vi "crc16-ccitt (xFFFF).vi"(8 "error in (no error)":errorcluster, 10 "Message":string) -> (0 "error out (dup)":errorcluster, 2 "CRC":u16 format="%.0x")   [LabVIEW 2017]
doc: "This VI takes in a string variable and calculates the 16-bit CRC value based on the CRC16-CCITT standard (polynomial 0x1021) with seed value of 0xFFFF ONLY!!!\n\nThis VI code is based on an extremely efficient implementation originally intended for microcontrollers and is adapted for LabVIEW. All thanks go to:\nOriginal Code: Ashley Roll\nOptimisations: Scott Dattalo"
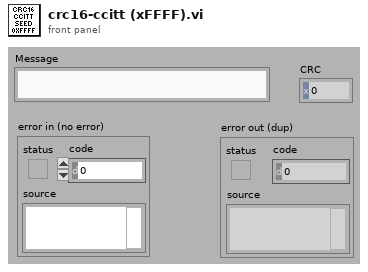
[diagram p1: front panel]
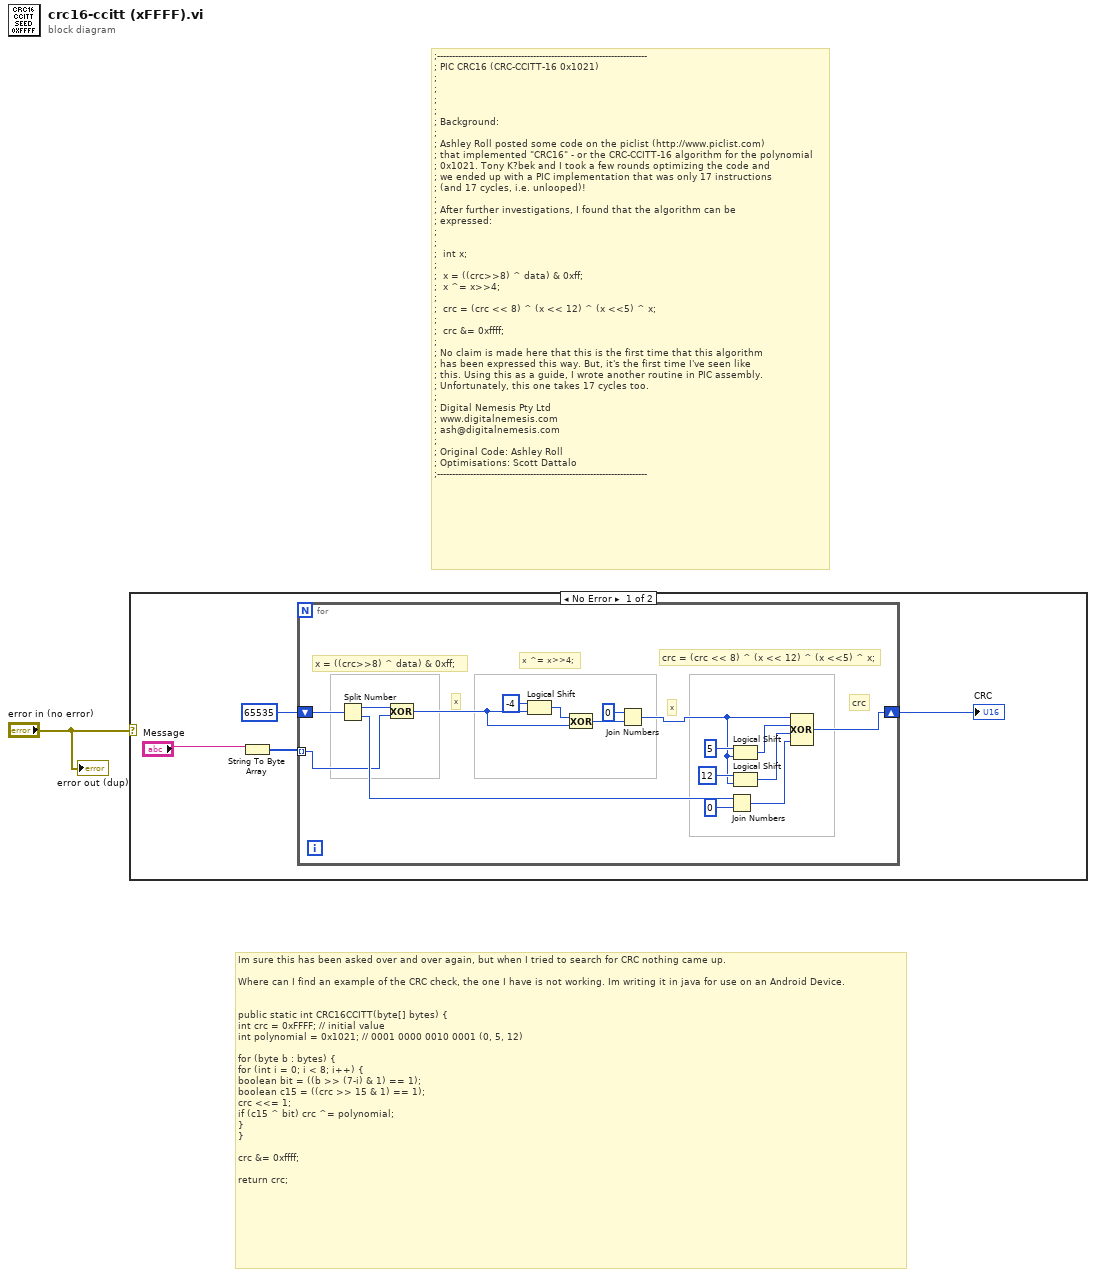
[diagram p0: block diagram]
diagram:
  # "Im sure this has been asked over and over again, but when I tried to search for CRC nothing came up.\n\nWhere can I find an example of the CRC check, the one I have is not working. Im writing it in java for use on an Android Device.\n\n\npublic static int CRC16CCITT(byte[] bytes) {\nint crc = 0xFFFF; // initial value\nint polynomial = 0x1021; // 0001 0000 0010 0001 (0, 5, 12) \n\nfor (byte b : bytes) {\nfor (int i = 0; i < 8; i++) {\nboolean bit = ((b >> (7-i) & 1) == 1);\nboolean c15 = ((crc >> 15 & 1) == 1);\ncrc <<= 1;\nif (c15 ^ bit) crc ^= polynomial;\n}\n}\n\ncrc &= 0xffff;\n\nreturn crc;"
  # ";----------------------------------------------------------------------\n; PIC CRC16 (CRC-CCITT-16 0x1021)\n;\n;\n; \n;\n; Background:\n;\n; Ashley Roll posted some code on the piclist (http://www.piclist.com)\n; that implemented \"CRC16\" - or the CRC-CCITT-16 algorithm for the polynomial\n; 0x1021. Tony K?bek and I took a few rounds optimizing the code and\n; we ended up with a PIC implementation that was only 17 instructions\n; (and 17 cycles, i.e. unlooped)!\n;\n; After further investigations, I found that the algorithm can be \n; expressed:\n;\n;\n;  int x;\n;\n;  x = ((crc>>8) ^ data) & 0xff;\n;  x ^= x>>4;\n;\n;  crc = (crc << 8) ^ (x << 12) ^ (x <<5) ^ x;\n;\n;  crc &= 0xffff;\n;\n; No claim is made here that this is the first time that this algorithm\n; has been expressed this way. But, it's the first time I've seen like\n; this. Using this as a guide, I wrote another routine in PIC assembly.\n; Unfortunately, this one takes 17 cycles too.\n;\n; Digital Nemesis Pty Ltd\n; www.digitalnemesis.com\n; ash@digitalnemesis.com\n;\n; Original Code: Ashley Roll\n; Optimisations: Scott Dattalo\n;----------------------------------------------------------------------"
  n1 = case shown="No Error" "error in (no error)" {
    frame No Error {
      n2 = String To Byte Array(string="Message") -> (unsigned byte array=w4:u8[])
      n3 = for {
        tunnel: w4 -> [w6] mode=indexing
        shift-right: [w12] -> w2
        shift-left: u16 65535 -> [w9]
        # "crc"
        # "crc = (crc << 8) ^ (x << 12) ^ (x <<5) ^ x;"
        # "x"
        # "x ^= x>>4;"
        # "x"
        # "x = ((crc>>8) ^ data) & 0xff;"
        n4 = Split Number(x=w9) -> (hi(x)=w7:u8, lo(x)=w14:u8)
        n5 = Exclusive Or(1:w6, 2:w7) -> (0:w11:u8)
        n6 = Logical Shift(y=i8 -4, x=w11) -> (x << y=w21:u8)
        n7 = Exclusive Or(1:w11, 2:w21) -> (0:w20:u8)
        n8 = Join Numbers(hi=u8 0, lo=w20) -> ((hi.lo)=w10:u16)
        n9 = Join Numbers(hi=w14, lo=u8 0) -> ((hi.lo)=w8:u16)
        n10 = Logical Shift(y=i8 5, x=w10) -> (x << y=w17:u16)
        n11 = Logical Shift(y=i8 12, x=w10) -> (x << y=w15:u16)
        n12 = Compound Arithmetic op=XOR(w10, w17, w15, w8) -> (w12:u16)
      }
      "CRC" <- w2
    }
    frame Error {
    }
  }
  "error out (dup)" <- "error in (no error)"
